vi "Display_LookUpTitleRGB.vi"(1 "ActivePixel":T1) -> (15 "Red":bool, 16 "Green":bool, 17 "Blue":bool)   [LabVIEW 2018]
uses:
  TypDefs/ActivePixel_Cluster.ctl
  <vilib>/rvi/DataTransferAndStorage/Container/Common/niFpgaContainerExecOnDevCompGetState.vi
  <vilib>/rvi/Emulation/niFpgaEmulationIsFPGAContextNoSignature.vi
  <vilib>/rvi/DataTransferAndStorage/Container/Common/niFpgaContainerGetUniqueNameForEmu.vi
  <vilib>/rvi/Emulation/niFpgaProcessEmulError.vi
  <vilib>/rvi/Emulation/niFpgaSctlEmulationGetInTimedLoop.vi
  <vilib>/rvi/errors/nirviReportUnexpectedCaseInternalError (U32).vi
  <vilib>/rvi/Memory/Memory_Emulation/niFpgaMemoryEmulationCacheClearOnFirstRun.vi
  <vilib>/rvi/Memory/Memory_Emulation/nirvimemoryEmulationManagerCache_MakeExclusive.vi
  <vilib>/rvi/Memory/Memory_Emulation/niFpgaMemoryEmulationValidateCache.vi
  <vilib>/rvi/Memory/Memory_Emulation/nirvimemoryEmulationManagerCache_InsertValue.vi
  <vilib>/Utility/error.llb/Clear Errors.vi
  <vilib>/rvi/Memory/Memory_Emulation/nirvimemoryEmulationManagerCache_ReleaseExclusive.vi
  <vilib>/rvi/Memory/Memory_Emulation/nirvimemoryEmulationManagerCache_GetValue.vi
  <vilib>/rvi/Memory/Memory_Emulation/nirvimemoryEmulationManagerCache_SetValue.vi
  <vilib>/rvi/Emulation/niFpgaSctlEmulationResourceMgr.vi
  <vilib>/rvi/DataTransferAndStorage/Container/XNode/niFpgaContainer.xnode
  <vilib>/rvi/Memory/Memory_Emulation/niFpgaMemoryEmulationRefIn.vi
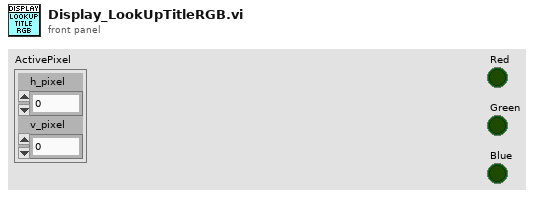
[diagram p1: front panel]
types:
  T1 = typedef "ActivePixel_Cluster.ctl" = cluster{"h_pixel":i16, "v_pixel":i16}
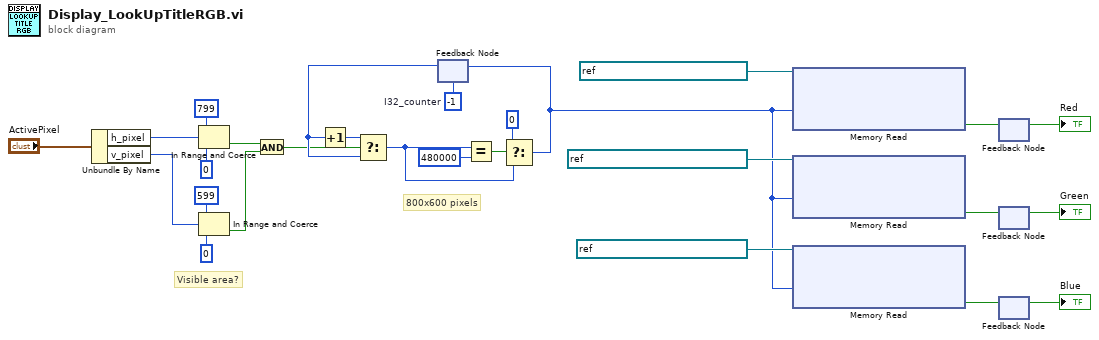
[diagram p0: block diagram]
diagram:
  w15 = -1  # I32_counter
  # "800x600 pixels"
  # "Visible area?"
  n1 = Unbundle By Name("ActivePixel") -> ("h_pixel"=w3:i16, "v_pixel"=w4:i16)
  n2 = In Range and Coerce(upper limit=i16 799, x=w3, lower limit=i16 0) -> (In Range?=w8:bool)  [unwired: 1 out]
  n3 = In Range and Coerce(upper limit=i16 599, x=w4, lower limit=i16 0) -> (In Range?=w5:bool)  [unwired: 1 out]
  n4 = And(x=w8, y=w5) -> (x .and. y?=w1:bool)
  n5 = feedback #1(w15) -> (w17:i32)
  n6 = Increment(x=w17) -> (x+1=w16:i32)
  n7 = Select(t=w16, s=w1, f=w17) -> (s? t:f=w18:i32)
  n8 = Equal?(x=w18, y=480000) -> (x = y?=w12:bool)
  n9 = Select(t=0, s=w12, f=w18) -> (s? t:f=w11:i32)
  n10 = feedback-in #1(w11) -> ()
  n11 = xnode ("Memory Read")("Address"=w11, "Memory In"=refnum<k21> "BlockMem_TitleScreenRed") -> ("Data"=w23:bool)  [unwired: 1 out]
  n12 = xnode ("Memory Read")("Address"=w11, "Memory In"=refnum<k21> "BlockMem_TitleScreenGreen") -> ("Data"=w22:bool)  [unwired: 1 out]
  n13 = xnode ("Memory Read")("Address"=w11, "Memory In"=refnum<k21> "BlockMem_TitleScreenBlue") -> ("Data"=w19:bool)  [unwired: 1 out]
  n14 = feedback #2() -> (→"Red":bool)  [unwired: 1 in]
  n15 = feedback-in #2(w23) -> ()
  n16 = feedback #3() -> (→"Green":bool)  [unwired: 1 in]
  n17 = feedback-in #3(w22) -> ()
  n18 = feedback #4() -> (→"Blue":bool)  [unwired: 1 in]
  n19 = feedback-in #4(w19) -> ()
